vi "MakeRoom.vi"(8 "error in (no error)":errorcluster, 10 "RoomNumber":i32, 11 "MazeGame in":refnum<class "MazeGame.lvclass">) -> (0 "error out":errorcluster, 2 "Room":refnum<class "Room.lvclass">, 3 "MazeGame out":refnum<class "MazeGame.lvclass">)   [LabVIEW 2020, in "FactoryMethod.lvlib" / "NoParametrizedFactoryMethod.lvlib" / "MazeGame.lvclass"]
uses:
  MazeGame.lvclass
  GoFcommonClasses/ConcreteMazeSite/Room/Room.lvclass
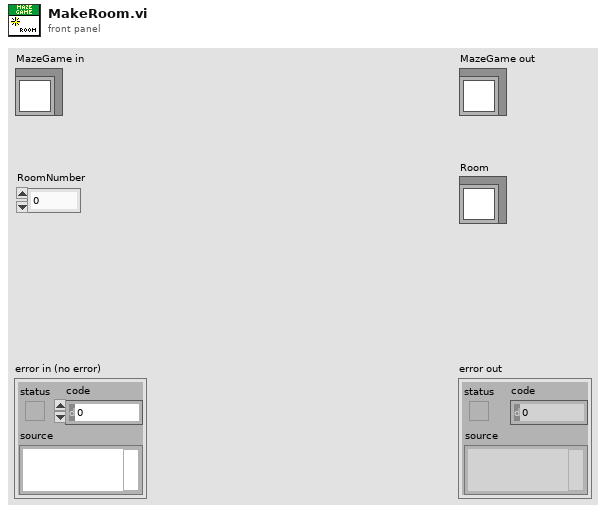
[diagram p1: front panel]
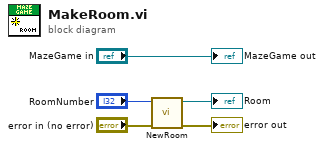
[diagram p0: block diagram]
diagram:
  n1 = call "NewRoom.vi"("error in (no error)"="error in (no error)", "RoomNumber"="RoomNumber") -> ("error out"=→"error out":errorcluster, "Room"=→"Room":refnum<class "Room.lvclass">)  [unwired: 8 in]
  "MazeGame out" <- "MazeGame in"
